vi "AllStage_Limits.vi"(8 "Axis":bool[](array[boolean])=[TRUE, TRUE, TRUE], 9 "Step(um)/Position(units)":dbl, 10 "Stage ID":string, 11 "MOVE/MVR":enum16{"MOVE", "MVR"}(ring)=enum."MVR") -> (0 "Positions":dbl[](array[numeric]), 1 "Boolean Array":bool[](array[boolean]), 2 "Stage ID":string)   [LabVIEW 2011]
panel:
  in  "Stage Array":T1(array[cluster])=[{"Upper"=10000.0, "Lower"=-10000.0, "UnitMult"=10.0, "ID"="ASI"}, {"Upper"=14.0, "Lower"=10.5, "UnitMult"=0.001, "ID"="M686"}, {"Upper"=1.0, "Lower"=-1.0, "UnitMult"=0.001, "ID"="M227"}, {"Upper"=100.0, "Lower"=0.0, "UnitMult"=1.0, "ID"="P612"}, {"Upper"=100.0, "Lower"=0.0, "UnitMult"=1.0, "ID"="P541"}, {"Upper"=15.0, "Lower"=0.0, "UnitMult"=0.001, "ID"="N664"}]
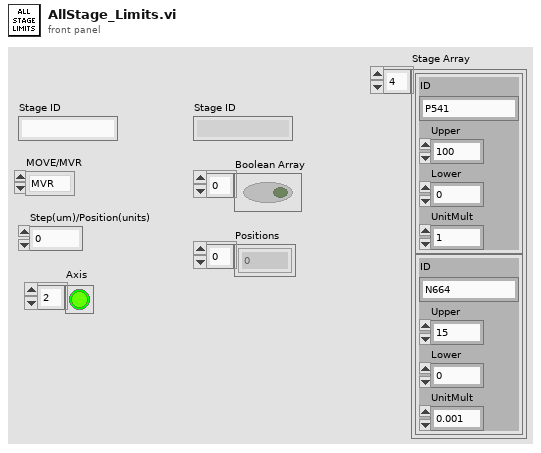
[diagram p1: front panel]
types:
  T1 = cluster{"Upper":dbl, "Lower":dbl, "UnitMult":dbl, "ID":string}[]
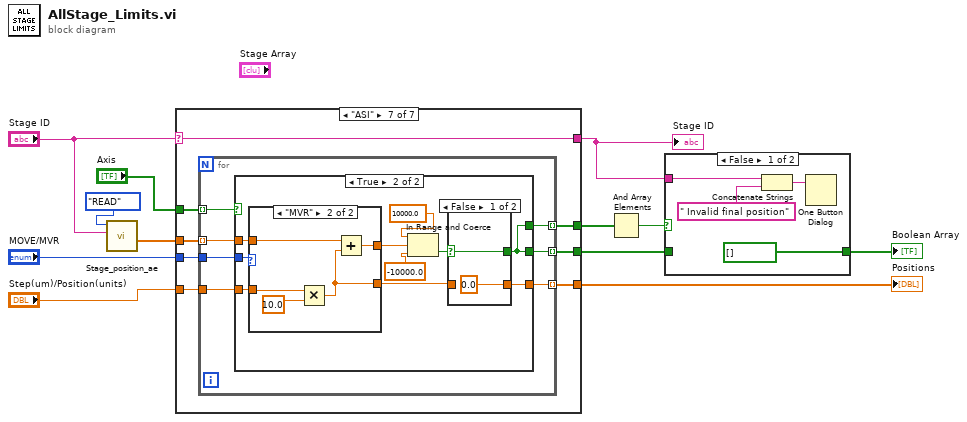
[diagram p0: block diagram]
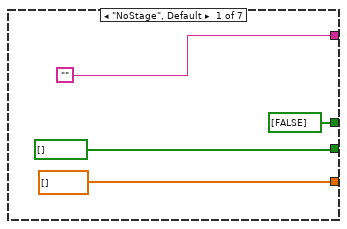
[diagram p3: hidden frame]
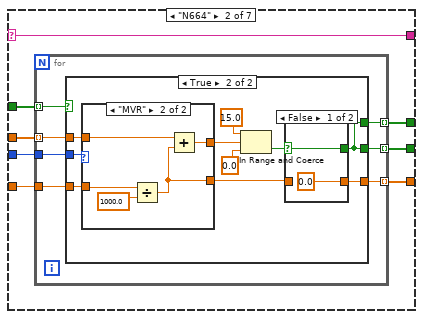
[diagram p4: hidden frame]
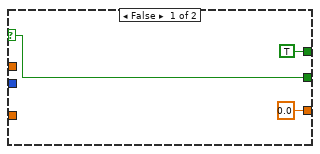
[diagram p5: hidden frame]
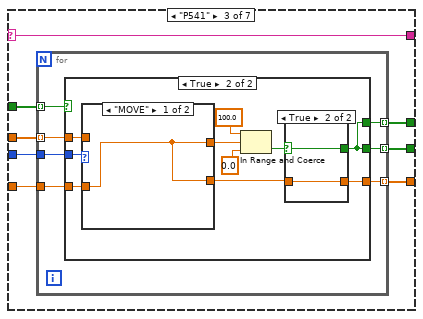
[diagram p8: hidden frame]
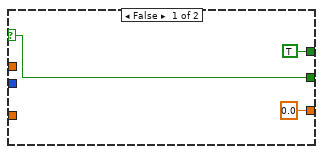
[diagram p9: hidden frame]
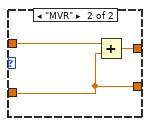
[diagram p10: hidden frame]
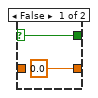
[diagram p11: hidden frame]
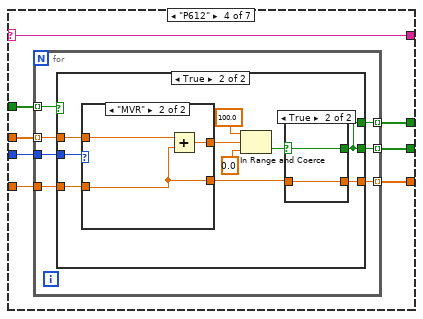
[diagram p12: hidden frame]
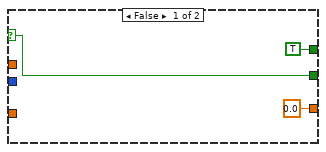
[diagram p13: hidden frame]
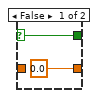
[diagram p15: hidden frame]
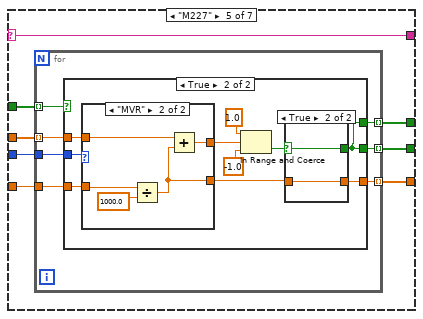
[diagram p16: hidden frame]
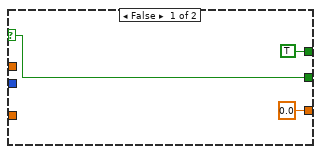
[diagram p17: hidden frame]
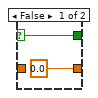
[diagram p19: hidden frame]
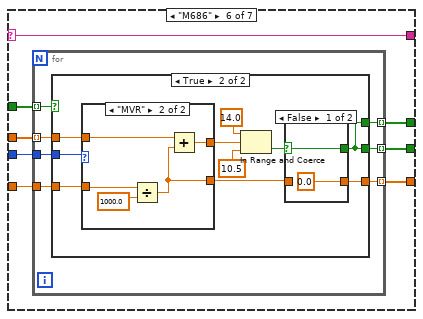
[diagram p20: hidden frame]
diagram:
  n1 = call "Stage_position_ae.vi"("StageID"="Stage ID", "Enum"=enum16{"WRITE", "READ"}."READ") -> ("Position Out"=w7:dbl[])  [unwired: 9 in]
  n2 = case shown="\"ASI\"" "Stage ID" {
    selector: "Stage ID" -> [_ w21 w57 w95 w131 w169 w207]
    tunnel: w7 -> [_ w22 w60 w96 w132 w170 w208]
    tunnel: ["" w21 w57 w95 w131 w169 w207] -> w3
    tunnel: "Step(um)/Position(units)" -> [_ w24 w62 w98 w134 w172 w210]
    tunnel: [bool[] [] w19 w58 w93 w129 w167 w205] -> w5
    tunnel: [dbl[] [] w23 w61 w97 w133 w171 w209] -> w12
    tunnel: "MOVE/MVR" -> [_ w20 w59 w94 w130 w168 w206]
    tunnel: "Axis" -> [_ w18 w56 w92 w128 w166 w204]
    tunnel: [bool[] [FALSE] w17 w55 w91 w127 w165 w203] -> w1
    frame "NoStage", Default {
    }
    frame "N664" {
      n3 = for {
        tunnel: w24 -> [w31]
        tunnel: [w28] -> w23 mode=indexing
        tunnel: w22 -> [w30] mode=indexing
        tunnel: [w29] -> w19 mode=indexing
        tunnel: w20 -> [w27]
        tunnel: w18 -> [w26] mode=indexing
        tunnel: [w25] -> w17 mode=indexing
        n4 = case shown="True" w26 {
          selector: w26 -> [w33 _]
          tunnel: w31 -> [_ w44]
          tunnel: w30 -> [_ w38]
          tunnel: [w33 w35] -> w29
          tunnel: [0.0 ("Step(um)/Position(units)") w37] -> w28
          tunnel: w27 -> [_ w36]
          tunnel: [TRUE w35] -> w25
          frame False {
          }
          frame True {
            n5 = case shown="\"MVR\"" w36 {
              tunnel: w44 -> [w45 w49]
              tunnel: [w45 w48] -> w43
              tunnel: [w45 w47] -> w40
              tunnel: w38 -> [_ w46]
              frame "MOVE" {
              }
              frame "MVR" {
                n6 = Divide(x=w49, y=1000.0) -> (x/y=w47:dbl)
                n7 = Add(x=w46, y=w47) -> (x+y=w48:dbl)
              }
            }
            n8 = In Range and Coerce(upper limit=15.0, x=w43, lower limit=0.0) -> (In Range?=w39:bool)  [unwired: 1 out]
            n9 = case shown="False" w39 {
              selector: w39 -> [w52 w54]
              tunnel: w40 -> [_ w53]
              tunnel: [w52 w54] -> w35
              tunnel: [0.0 w53] -> w37
              frame False {
              }
              frame True {
              }
            }
          }
        }
      }
    }
    frame "P541" {
      n10 = for {
        tunnel: w62 -> [w69]
        tunnel: [w66] -> w61 mode=indexing
        tunnel: w60 -> [w68] mode=indexing
        tunnel: [w67] -> w58 mode=indexing
        tunnel: w59 -> [w65]
        tunnel: w56 -> [w64] mode=indexing
        tunnel: [w63] -> w55 mode=indexing
        n11 = case shown="True" w64 {
          selector: w64 -> [w71 _]
          tunnel: w69 -> [_ w82]
          tunnel: w68 -> [_ w76]
          tunnel: [w71 w73] -> w67
          tunnel: [0.0 ("Step(um)/Position(units)") w75] -> w66
          tunnel: w65 -> [_ w74]
          tunnel: [TRUE w73] -> w63
          frame False {
          }
          frame True {
            n12 = case shown="\"MOVE\"" w74 {
              tunnel: w82 -> [w83 w84]
              tunnel: [w83 w86] -> w81
              tunnel: [w83 w84] -> w78
              tunnel: w76 -> [_ w85]
              frame "MOVE" {
              }
              frame "MVR" {
                n13 = Add(x=w85, y=w84) -> (x+y=w86:dbl)
              }
            }
            n14 = In Range and Coerce(upper limit=100.0, x=w81, lower limit=0.0) -> (In Range?=w77:bool)  [unwired: 1 out]
            n15 = case shown="True" w77 {
              selector: w77 -> [w88 w90]
              tunnel: w78 -> [_ w89]
              tunnel: [w88 w90] -> w73
              tunnel: [0.0 w89] -> w75
              frame False {
              }
              frame True {
              }
            }
          }
        }
      }
    }
    frame "P612" {
      n16 = for {
        tunnel: w98 -> [w105]
        tunnel: [w102] -> w97 mode=indexing
        tunnel: w96 -> [w104] mode=indexing
        tunnel: [w103] -> w93 mode=indexing
        tunnel: w94 -> [w101]
        tunnel: w92 -> [w100] mode=indexing
        tunnel: [w99] -> w91 mode=indexing
        n17 = case shown="True" w100 {
          selector: w100 -> [w108 _]
          tunnel: w105 -> [_ w118]
          tunnel: w104 -> [_ w112]
          tunnel: [w108 w109] -> w103
          tunnel: [0.0 ("Step(um)/Position(units)") w111] -> w102
          tunnel: w101 -> [_ w110]
          tunnel: [TRUE w109] -> w99
          frame False {
          }
          frame True {
            n18 = case shown="\"MVR\"" w110 {
              tunnel: w118 -> [w119 w120]
              tunnel: [w119 w122] -> w117
              tunnel: [w119 w120] -> w114
              tunnel: w112 -> [_ w121]
              frame "MOVE" {
              }
              frame "MVR" {
                n19 = Add(x=w121, y=w120) -> (x+y=w122:dbl)
              }
            }
            n20 = In Range and Coerce(upper limit=100.0, x=w117, lower limit=0.0) -> (In Range?=w113:bool)  [unwired: 1 out]
            n21 = case shown="True" w113 {
              selector: w113 -> [w124 w126]
              tunnel: w114 -> [_ w125]
              tunnel: [w124 w126] -> w109
              tunnel: [0.0 w125] -> w111
              frame False {
              }
              frame True {
              }
            }
          }
        }
      }
    }
    frame "M227" {
      n22 = for {
        tunnel: w134 -> [w141]
        tunnel: [w138] -> w133 mode=indexing
        tunnel: w132 -> [w140] mode=indexing
        tunnel: [w139] -> w129 mode=indexing
        tunnel: w130 -> [w137]
        tunnel: w128 -> [w136] mode=indexing
        tunnel: [w135] -> w127 mode=indexing
        n23 = case shown="True" w136 {
          selector: w136 -> [w143 _]
          tunnel: w141 -> [_ w154]
          tunnel: w140 -> [_ w148]
          tunnel: [w143 w145] -> w139
          tunnel: [0.0 ("Step(um)/Position(units)") w147] -> w138
          tunnel: w137 -> [_ w146]
          tunnel: [TRUE w145] -> w135
          frame False {
          }
          frame True {
            n24 = case shown="\"MVR\"" w146 {
              tunnel: w154 -> [w155 w159]
              tunnel: [w155 w158] -> w153
              tunnel: [w155 w157] -> w150
              tunnel: w148 -> [_ w156]
              frame "MOVE" {
              }
              frame "MVR" {
                n25 = Divide(x=w159, y=1000.0) -> (x/y=w157:dbl)
                n26 = Add(x=w156, y=w157) -> (x+y=w158:dbl)
              }
            }
            n27 = In Range and Coerce(upper limit=1.0, x=w153, lower limit=-1.0) -> (In Range?=w149:bool)  [unwired: 1 out]
            n28 = case shown="True" w149 {
              selector: w149 -> [w162 w164]
              tunnel: w150 -> [_ w163]
              tunnel: [w162 w164] -> w145
              tunnel: [0.0 w163] -> w147
              frame False {
              }
              frame True {
              }
            }
          }
        }
      }
    }
    frame "M686" {
      n29 = for {
        tunnel: w172 -> [w179]
        tunnel: [w176] -> w171 mode=indexing
        tunnel: w170 -> [w178] mode=indexing
        tunnel: [w177] -> w167 mode=indexing
        tunnel: w168 -> [w175]
        tunnel: w166 -> [w174] mode=indexing
        tunnel: [w173] -> w165 mode=indexing
        n30 = case shown="True" w174 {
          selector: w174 -> [w182 _]
          tunnel: w179 -> [_ w192]
          tunnel: w178 -> [_ w186]
          tunnel: [w182 w183] -> w177
          tunnel: [0.0 ("Step(um)/Position(units)") w185] -> w176
          tunnel: w175 -> [_ w184]
          tunnel: [TRUE w183] -> w173
          frame False {
          }
          frame True {
            n31 = case shown="\"MVR\"" w184 {
              tunnel: w192 -> [w193 w197]
              tunnel: [w193 w196] -> w191
              tunnel: [w193 w195] -> w188
              tunnel: w186 -> [_ w194]
              frame "MOVE" {
              }
              frame "MVR" {
                n32 = Divide(x=w197, y=1000.0) -> (x/y=w195:dbl)
                n33 = Add(x=w194, y=w195) -> (x+y=w196:dbl)
              }
            }
            n34 = In Range and Coerce(upper limit=14.0, x=w191, lower limit=10.5) -> (In Range?=w187:bool)  [unwired: 1 out]
            n35 = case shown="False" w187 {
              selector: w187 -> [w200 w202]
              tunnel: w188 -> [_ w201]
              tunnel: [w200 w202] -> w183
              tunnel: [0.0 w201] -> w185
              frame False {
              }
              frame True {
              }
            }
          }
        }
      }
    }
    frame "ASI" {
      n36 = for {
        tunnel: w210 -> [w217]
        tunnel: [w214] -> w209 mode=indexing
        tunnel: w208 -> [w216] mode=indexing
        tunnel: [w215] -> w205 mode=indexing
        tunnel: w206 -> [w213]
        tunnel: w204 -> [w212] mode=indexing
        tunnel: [w211] -> w203 mode=indexing
        n37 = case shown="True" w212 {
          selector: w212 -> [w220 _]
          tunnel: w217 -> [_ w230]
          tunnel: w216 -> [_ w224]
          tunnel: [w220 w221] -> w215
          tunnel: [0.0 ("Step(um)/Position(units)") w223] -> w214
          tunnel: w213 -> [_ w222]
          tunnel: [TRUE w221] -> w211
          frame False {
          }
          frame True {
            n38 = case shown="\"MVR\"" w222 {
              tunnel: w230 -> [w231 w235]
              tunnel: [w231 w234] -> w229
              tunnel: [w231 w233] -> w226
              tunnel: w224 -> [_ w232]
              frame "MOVE" {
              }
              frame "MVR" {
                n39 = Multiply(x=w235, y=10.0) -> (x*y=w233:dbl)
                n40 = Add(x=w232, y=w233) -> (x+y=w234:dbl)
              }
            }
            n41 = In Range and Coerce(upper limit=10000.0, x=w229, lower limit=-10000.0) -> (In Range?=w225:bool)  [unwired: 1 out]
            n42 = case shown="False" w225 {
              selector: w225 -> [w238 w240]
              tunnel: w226 -> [_ w239]
              tunnel: [w238 w240] -> w221
              tunnel: [0.0 w239] -> w223
              frame False {
              }
              frame True {
              }
            }
          }
        }
      }
    }
  }
  "Positions" <- w12
  "Stage ID" <- w3
  n43 = And Array Elements(Boolean array=w1) -> (logical AND=w6:bool)
  n44 = case shown="False" w6 {
    tunnel: [bool[] [] w245] -> w4
    tunnel: w5 -> [_ w245]
    tunnel: w3 -> [w241 _]
    frame False {
      n45 = Concatenate Strings(w241, " Invalid final position") -> (w244:string)
      n46 = One Button Dialog(message=w244) -> ()  [unwired: 1 in, 1 out]
    }
    frame True {
    }
  }
  "Boolean Array" <- w4
